vi "Msg To.vi"(10 "String Indicator":string) -> (3 "String Indicator Event out":refnum<class "String Indicator Msg.lvclass">)   [LabVIEW 2021, in "String Indicator.lvlib" / "String Indicator Msg.lvclass"]
uses:
  String Indicator Msg.lvclass
  String Indicator Msg.lvclass/String Indicator Msg.ctl
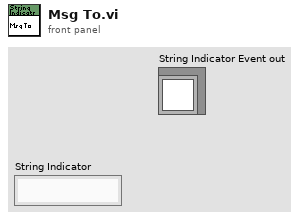
[diagram p1: front panel]
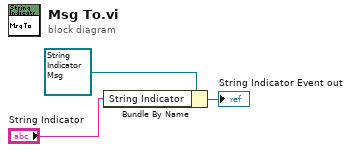
[diagram p0: block diagram]
diagram:
  n1 = Bundle By Name(cluster=refnum<class "String Indicator Msg.lvclass"> refnum ("String Indicator Ref.lvlib:String Indicator Msg.lvclass"), "String Indicator"="String Indicator") -> (→"String Indicator Event out":refnum<class "String Indicator Msg.lvclass">)
